vi "Disk Drive Serial Numbers Using .Net.vi"(8 "error in":errorcluster) -> (0 "error out":errorcluster, 2 "Serial Numbers Decoded":string[](array[string]), 3 "Serial Numbers":string[](array[string]))   [LabVIEW 2021]
uses:
  System.Management
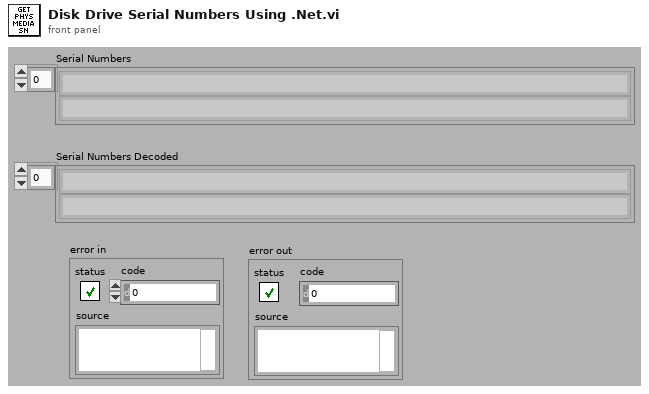
[diagram p1: front panel]
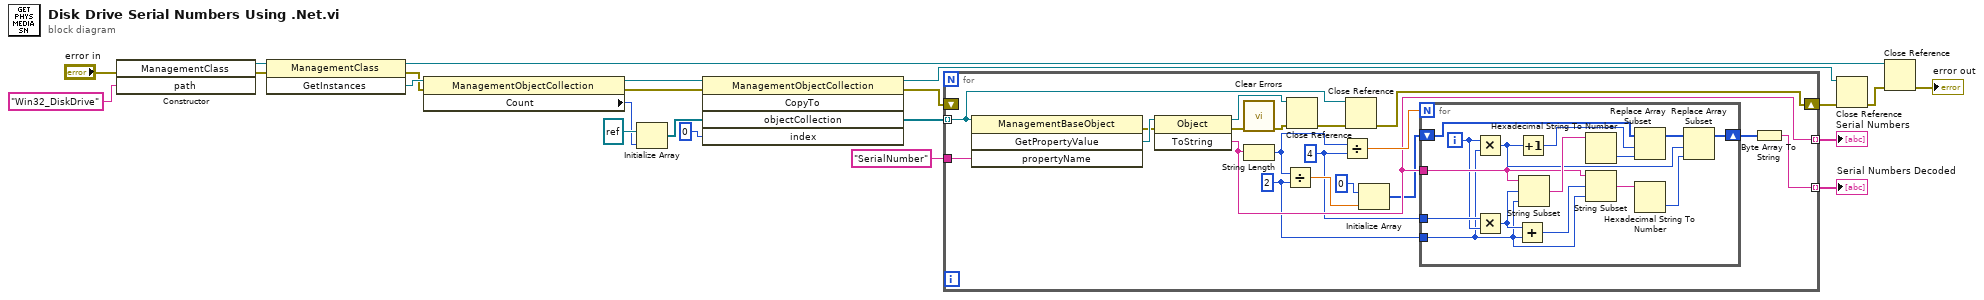
[diagram p0: block diagram]
diagram:
  n1 = constructor class="ManagementClass"(error in="error in", "path"="Win32_DiskDrive") -> (reference out=w21:refnum<k24>, error out=w14:errorcluster)  [unwired: 2 in, 2 out]
  n2 = invoke class="ManagementClass" method="GetInstances"(reference=w21, error in=w14) -> (reference out=w12:refnum<k24>, error out=w11:errorcluster, "GetInstances"=w19:refnum<k24>)  [unwired: 1 in]
  n3 = property class="ManagementObjectCollection"(reference=w19, error in=w11) -> (reference out=w10:refnum<k24>, error out=w9:errorcluster, "Count"=w18:i32)
  n4 = Initialize Array(refnum<k24> refnum, w18) -> (w17:refnum<k24>[])
  n5 = invoke class="ManagementObjectCollection" method="CopyTo"(reference=w10, error in=w9, "objectCollection"=w17, "index"=0) -> (reference out=w7:refnum<k24>, error out=w6:errorcluster, "objectCollection"=w15:refnum<k24>[])  [unwired: 1 in, 2 out]
  n6 = for {
    tunnel: w15 -> [w36] mode=indexing
    tunnel: "SerialNumber" ("propertyName") -> [w34]
    shift-right: [w39] -> w5
    shift-left: w6 -> [_]
    tunnel: [w31] -> w2 mode=indexing
    tunnel: [w30] -> w1 mode=indexing
    w24 = 4 ("y")
    w23 = 2 ("y")
    n7 = invoke class="ManagementBaseObject" method="GetPropertyValue"(reference=w36, "propertyName"=w34) -> (error out=w37:errorcluster, "GetPropertyValue"=w38:refnum<k24>)  [unwired: 2 in, 2 out]
    n8 = invoke class="Object" method="ToString"(reference=w38, error in=w37) -> (reference out=w35:refnum<k24>, error out=w41:errorcluster, "ToString"=w31:string)  [unwired: 1 in]
    n9 = call <vilib>:"Clear Errors.vi"("error in (no error)"=w41) -> ("error out"=w33:errorcluster)  [unwired: 5 in, 1 out]
    n10 = String Length(string=w31) -> (length=w29:i32)
    n11 = Divide(x=w29, y=w23) -> (x/y=w28:dbl)
    n12 = Close Reference(reference=w35, error in (no error)=w33) -> (error out=w40:errorcluster)
    n13 = Divide(x=w29, y=w24) -> (x/y=w32:dbl)
    n14 = Close Reference(reference=w36, error in (no error)=w40) -> (error out=w39:errorcluster)
    n15 = Initialize Array(u8 0 ("y"), w28) -> (w26:u8[])
    n16 = for {
      N: w32 -> [_]
      tunnel: w31 -> [w48]
      tunnel: w24 -> [w54]
      shift-right: [w51] -> w25
      shift-left: w26 -> [w53]
      tunnel: w23 -> [w43]
      i -> [w44]
      n17 = Multiply(x=w44, y=w43) -> (x*y=w42:i32)
      n18 = Multiply(x=w54, y=w44) -> (x*y=w46:i32)
      n19 = Add(x=w46, y=w43) -> (x+y=w45:i32)
      n20 = Increment(x=w42) -> (x+1=w47:i32)
      n21 = String Subset(string=w48, offset (0)=w46, length (rest)=w43) -> (substring=w56:string)
      n22 = Hexadecimal String To Number(string=w56) -> (number=w50:u32)  [unwired: 2 in, 1 out]
      n23 = String Subset(string=w48, offset (0)=w45, length (rest)=w43) -> (substring=w55:string)
      n24 = Replace Array Subset(array=w53, new element=w50, index=w47) -> (w52:u8[])
      n25 = Hexadecimal String To Number(string=w55) -> (number=w49:u32)  [unwired: 2 in, 1 out]
      n26 = Replace Array Subset(array=w52, new element=w49, index=w42) -> (w51:u8[])
    }
    n27 = Byte Array To String(unsigned byte array=w25) -> (string=w30:string)
  }
  "Serial Numbers" <- w2
  "Serial Numbers Decoded" <- w1
  n28 = Close Reference(reference=w7, error in (no error)=w5) -> (error out=w8:errorcluster)
  n29 = Close Reference(reference=w12, error in (no error)=w8) -> (error out=→"error out":errorcluster)
